vi "Counter_once.vi"(10 "reset":bool, 11 "limit":u16) -> (3 "count":u16)   [LabVIEW 2017]
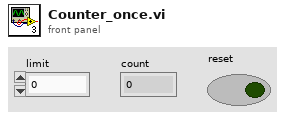
[diagram p1: front panel]
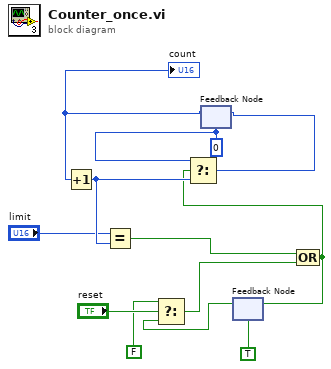
[diagram p0: block diagram]
diagram:
  w6 = u16 0
  n1 = feedback #1(w6) -> (w5:u16)
  "count" <- w5
  n2 = Increment(x=w5) -> (x+1=w11:u16)
  n3 = Equal?(x="limit", y=w11) -> (x = y?=w9:bool)
  n4 = feedback #2(TRUE) -> (w2:bool)
  n5 = Select(t=FALSE, s="reset", f=w2) -> (s? t:f=w3:bool)
  n6 = Compound Arithmetic op=OR(w9, w3) -> (w8:bool)
  n7 = Select(t=w6, s=w8, f=w11) -> (s? t:f=w12:u16)
  n8 = feedback-in #1(w12) -> ()
  n9 = feedback-in #2(w8) -> ()
